vi "SQL Update Data.vi"(7 "Where Condition":string, 8 "error in":errorcluster, 9 "Set Data":T6, 10 "Table Name":string, 11 "Schema":string) -> (0 "error out":errorcluster, 3 "Query":string)   [LabVIEW 2023, in "HardwareAbstractionLayer_LVOOP.lvlib" / "Report.lvclass"]
uses:
  Report.lvclass
  Control/UUT Test Info.ctl
  Control/FE FRAME LOG.ctl
  Control/FF FRAME LOG.ctl
  Control/LIMIT TABLE.ctl
  Control/ERROR LOG.ctl
  Database/SQL Public VI/Control/DB Options.ctl
  Database/Database.lvclass
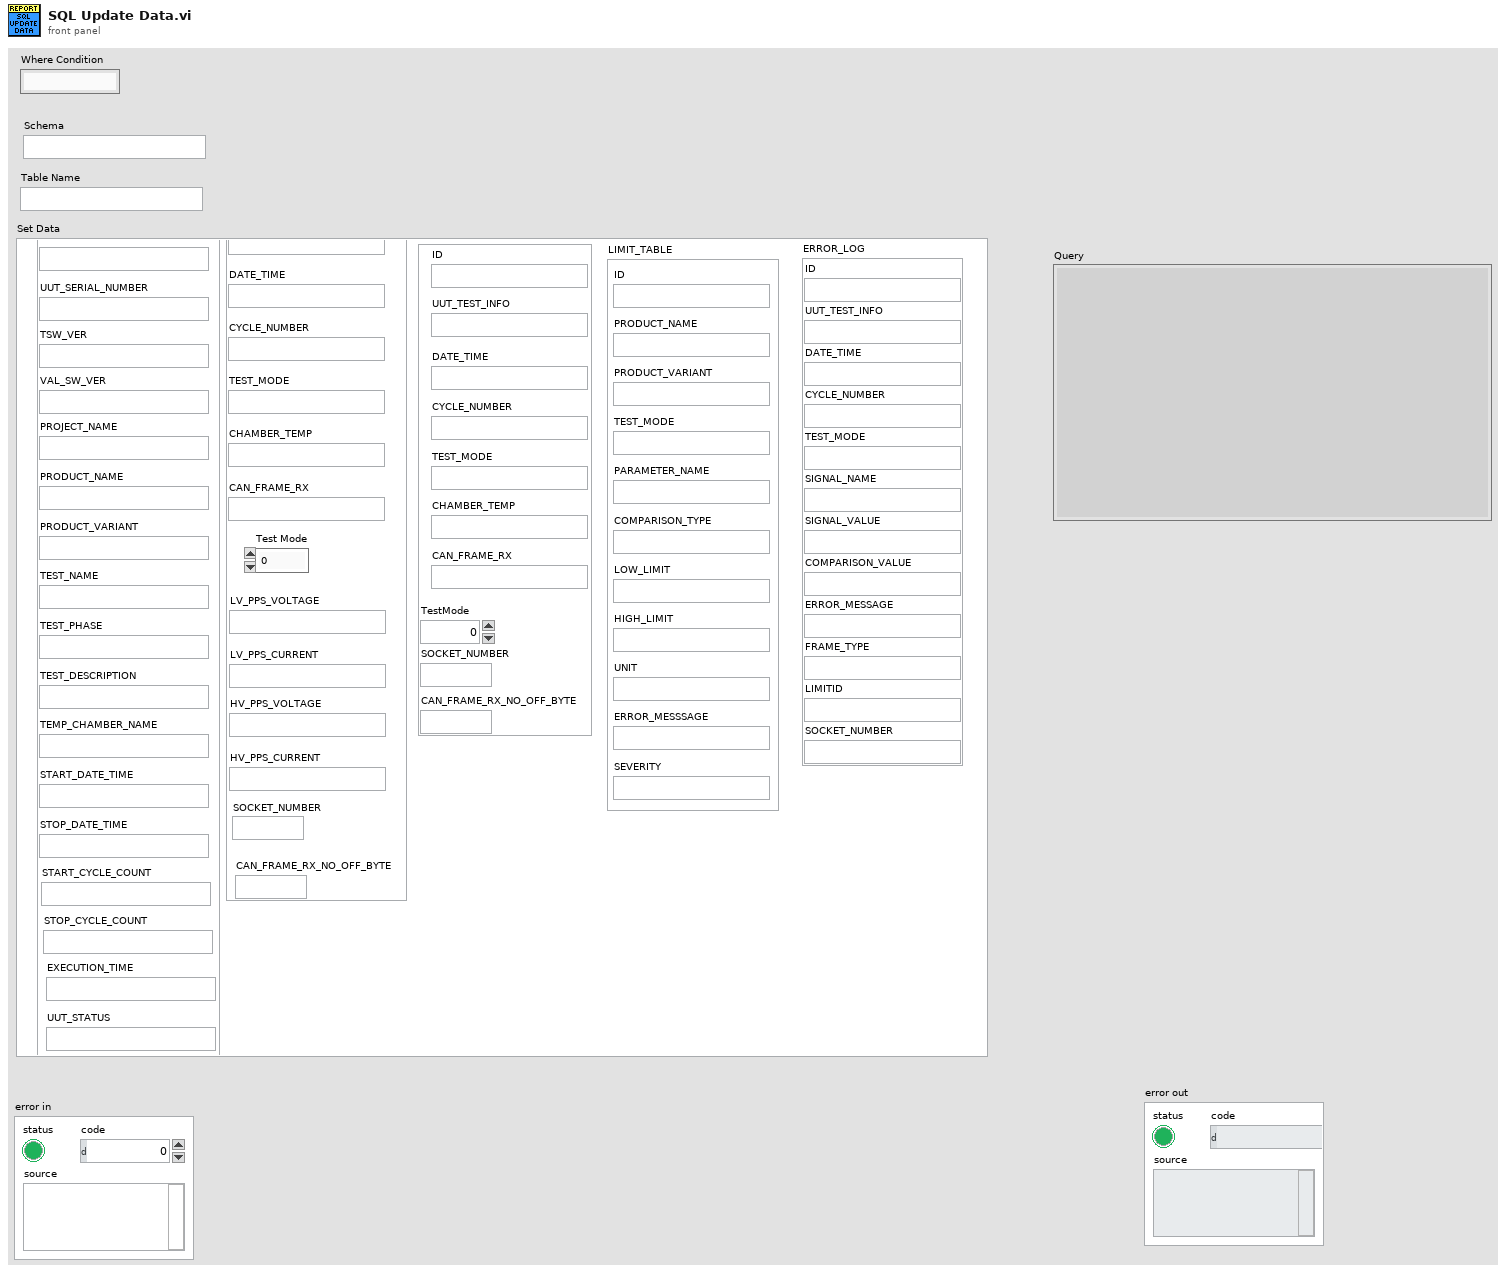
[diagram p1: front panel]
types:
  T1 = typedef "HardwareAbstractionLayer_LVOOP.lvlib/Report.lvclass/UUT Test Info.ctl" = cluster{"ID":string, "STATION_ID":string, "TEST_SOCKET_INDEX":string, "UUT_SERIAL_NUMBER":string, "TSW_VER":string, "VAL_SW_VER":string, "PROJECT_NAME":string, "PRODUCT_NAME":string, "PRODUCT_VARIANT":string, "TEST_NAME":string, "TEST_PHASE":string, "TEST_DESCRIPTION":string, "TEMP_CHAMBER_NAME":string, "START_DATE_TIME":string, "STOP_DATE_TIME ":string, "START_CYCLE_COUNT":string, "STOP_CYCLE_COUNT":string, "EXECUTION_TIME":string, "UUT_STATUS":string, "UUT_ERROR_CODE":string, "UUT_ERROR_MESSAGE":string, "TEST_SEQUENCE":string}
  T2 = typedef "HardwareAbstractionLayer_LVOOP.lvlib/Report.lvclass/FE FRAME LOG.ctl" = cluster{"ID":string, "UUT_TEST_INFO":string, "DATE_TIME":string, "CYCLE_NUMBER":string, "TEST_MODE":string, "CHAMBER_TEMP":string, "CAN_FRAME_RX":string, "Test Mode":u32, "LV_PPS_VOLTAGE":string, "LV_PPS_CURRENT":string, "HV_PPS_VOLTAGE":string, "HV_PPS_CURRENT":string, "SOCKET_NUMBER":string, "CAN_FRAME_RX_NO_OFF_BYTE":string}
  T3 = typedef "HardwareAbstractionLayer_LVOOP.lvlib/Report.lvclass/FF FRAME LOG.ctl" = cluster{"ID":string, "UUT_TEST_INFO":string, "DATE_TIME":string, "CYCLE_NUMBER":string, "TEST_MODE":string, "CAN_FRAME_RX":string, "CHAMBER_TEMP":string, "TestMode":u32, "SOCKET_NUMBER":string, "CAN_FRAME_RX_NO_OFF_BYTE":string}
  T4 = typedef "HardwareAbstractionLayer_LVOOP.lvlib/Report.lvclass/LIMIT TABLE.ctl" = cluster{"ID":string, "PRODUCT_NAME":string, "PRODUCT_VARIANT":string, "TEST_MODE":string, "PARAMETER_NAME":string, "COMPARISON_TYPE":string, "LOW_LIMIT":string, "HIGH_LIMIT":string, "UNIT":string, "ERROR_MESSSAGE":string, "SEVERITY":string}
  T5 = typedef "HardwareAbstractionLayer_LVOOP.lvlib/Report.lvclass/ERROR LOG.ctl" = cluster{"ID":string, "UUT_TEST_INFO":string, "DATE_TIME":string, "CYCLE_NUMBER":string, "TEST_MODE":string, "SIGNAL_NAME":string, "SIGNAL_VALUE":string, "COMPARISON_VALUE":string, "ERROR_MESSAGE":string, "FRAME_TYPE":string, "LIMITID":string, "SOCKET_NUMBER":string}
  T6 = cluster{"UUT_TEST_INFO":T1, "FE_FRAME_LOG":T2, "FF_FRAME_LOG":T3, "LIMIT_TABLE":T4, "ERROR_LOG":T5}
  T7 = typedef "HardwareAbstractionLayer_LVOOP.lvlib/Database.lvclass/DB Options.ctl" = enum16{"Init", "Select Data", "Insert Data", "Update Data", "Delete Data", "Execute Query", "Create Schema", "Create Table", "List Tables", "List Columns", "Close"}
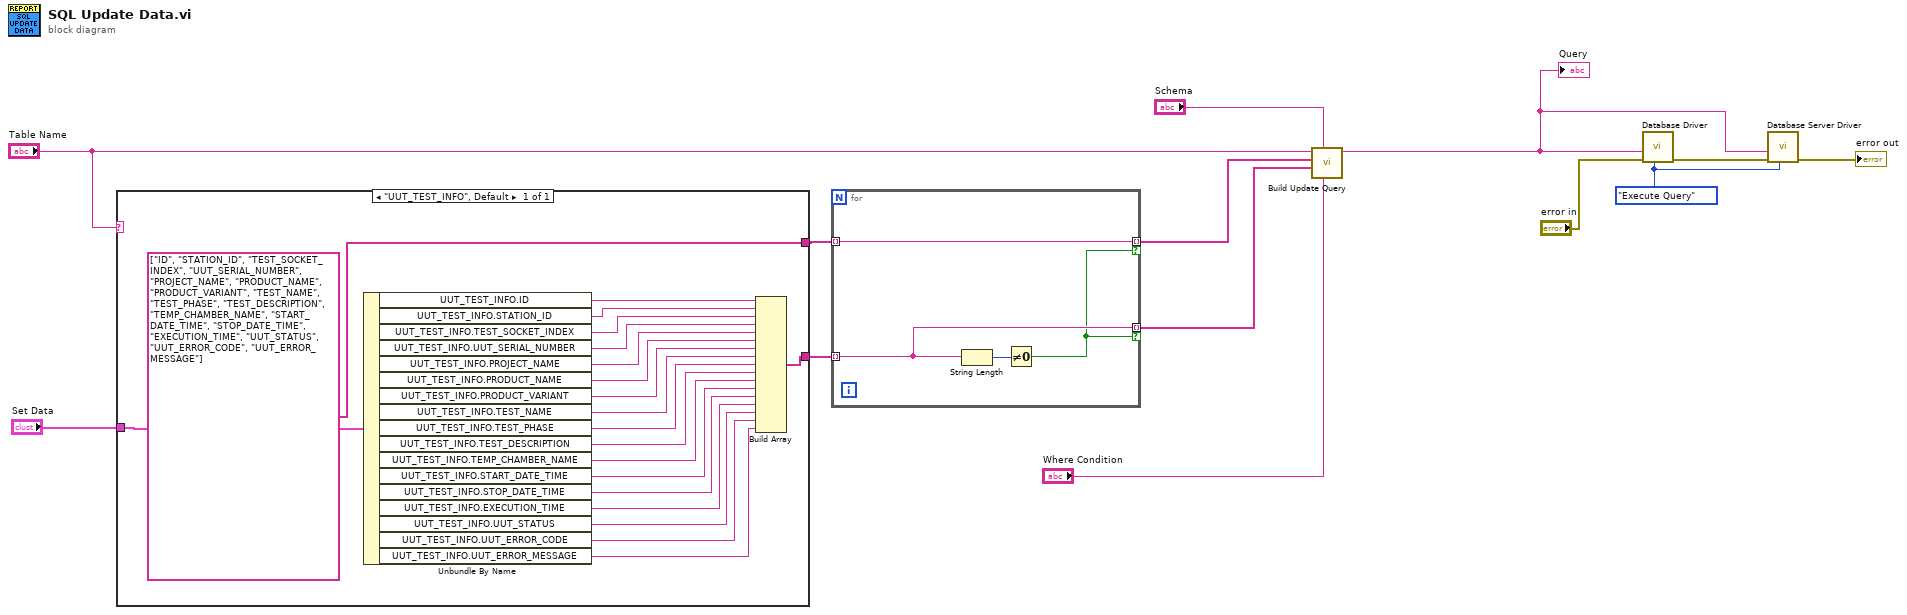
[diagram p0: block diagram]
diagram:
  w2 = DB_Options."Execute Query" ("Options")
  n1 = case shown="\"UUT_TEST_INFO\", Default" "Table Name" {
    tunnel: "Set Data" -> [w33]
    tunnel: [string[] ["ID", "STATION_ID", "TEST_SOCKET_INDEX", "UUT_SERIAL_NUMBER", "PROJECT_NAME", "PRODUCT_NAME", "PRODUCT_VARIANT", "TEST_NAME", "TEST_PHASE", "TEST_DESCRIPTION", "TEMP_CHAMBER_NAME", "START_DATE_TIME", "STOP_DATE_TIME", "EXECUTION_TIME", "UUT_STATUS", "UUT_ERROR_CODE", "UUT_ERROR_MESSAGE"] ("DB Column Name")] -> w12
    tunnel: [w16] -> w11
    frame "UUT_TEST_INFO", Default {
      n2 = Unbundle By Name(w33) -> ("UUT_TEST_INFO.ID"=w32:string, "UUT_TEST_INFO.STATION_ID"=w31:string, "UUT_TEST_INFO.TEST_SOCKET_INDEX"=w30:string, "UUT_TEST_INFO.UUT_SERIAL_NUMBER"=w29:string, "UUT_TEST_INFO.PROJECT_NAME"=w28:string, "UUT_TEST_INFO.PRODUCT_NAME"=w27:string, "UUT_TEST_INFO.PRODUCT_VARIANT"=w26:string, "UUT_TEST_INFO.TEST_NAME"=w25:string, "UUT_TEST_INFO.TEST_PHASE"=w24:string, "UUT_TEST_INFO.TEST_DESCRIPTION"=w23:string, "UUT_TEST_INFO.TEMP_CHAMBER_NAME"=w22:string, "UUT_TEST_INFO.START_DATE_TIME"=w21:string, "UUT_TEST_INFO.STOP_DATE_TIME"=w20:string, "UUT_TEST_INFO.EXECUTION_TIME"=w19:string, "UUT_TEST_INFO.UUT_STATUS"=w18:string, "UUT_TEST_INFO.UUT_ERROR_CODE"=w15:string, "UUT_TEST_INFO.UUT_ERROR_MESSAGE"=w14:string)
      n3 = Build Array(w32, w31, w30, w29, w28, w27, w26, w25, w24, w23, w22, w21, w20, w19, w18, w15, w14) -> (w16:string[])
    }
  }
  n4 = for {
    tunnel: w12 -> [w35] mode=indexing
    tunnel: w11 -> [w36] mode=indexing
    tunnel: [w36] -> w6 mode=indexing if=w34
    tunnel: [w35] -> w7 mode=indexing if=w34
    n5 = String Length(string=w36) -> (length=w37:i32)
    n6 = Not Equal To 0?(x=w37) -> (x != 0?=w34:bool)
  }
  n7 = call "Build Update Query.vi"("Where"="Where Condition", "Schema Name"="Schema", "Data"=w6, "Column Names"=w7, "Table Name"="Table Name") -> ("SQL"=w1:string)  [unwired: 5 in, 1 out]
  "Query" <- w1
  n8 = call "Database Driver.vi"("Options"=w2, "error in"="error in", "SQL query"=w1) -> ("error out"=w4:errorcluster)  [unwired: 5 in, 3 out]
  n9 = call "Database Server Driver.vi"("Options"=w2, "error in"=w4, "SQL query"=w1) -> ("error out"=→"error out":errorcluster)  [unwired: 5 in, 3 out]
